vi "Regler Ausgang.vi"(7 "Index":i32, 8 "Fehler":errorcluster caption="Fehler (Eingang)") -> (0 "Fehler (Ausgang)":errorcluster)   [LabVIEW 2020, in "Regler.lvlib" / "Druckregler.lvlib"]
uses:
  Druckregler.lvlib
  Aktionen Param. Druckregler.ctl
  Aktionen Interne Werte.ctl
  Allgemein/FGV Zustaende Aktionen.ctl
  Funktionstasten/Zustaende.ctl
  Allgemein/Aktionen FGV Dichtheitstest.ctl
  Allgemein/Aktion FGV Messbetrieb.ctl
  Verwaltung/FGV IN Aktionen.ctl
  Konfig-Dateien/FGV Betriebsdaten Aktionen.ctl
  Verwaltung/Verwaltung - cRIO.lvlib
  Allgemein/Allgemein.lvlib
  Konfig-Dateien/Konfig-Dateien.lvlib
  Regler.lvlib
  Funktionstasten/Funktionstasten.lvlib
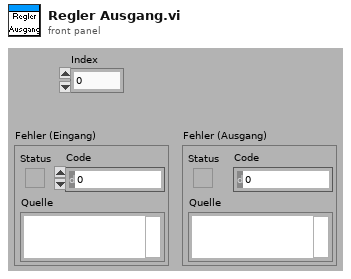
[diagram p1: front panel]
types:
  T1 = typedef "Allgemein.lvlib/Aktion FGV Messbetrieb.ctl" = enum16{"lesen", "schreiben"}
  T2 = typedef "Allgemein.lvlib/Aktionen FGV Dichtheitstest.ctl" = enum16{"lesen", "schreiben"}
  T3 = typedef "Funktionstasten.lvlib/Zustaende.ctl" = enum16{"Standby", "Pause", "Eco", "Messen", "Kalibrieren", "Spülen Filter", "Spülen Leitung", "Umgebungsluft", "0-Gas", "Cal-Gas", "CG zu PNS", "-------------", "Init 1", "Init 2", "Init 3", "Init 4", "Messen vorbereiten", "Messen durchführen", "Exit"}
  T4 = enum16{"Standby", "Pause", "Eco", "Messen", "Kalibrieren", "Spülen Filter", "Spülen Leitung", "Umgebungsluft", "0-Gas", "Cal-Gas 1", "CG zu PNS", "-------------", "Init 1", "Init 2", "Init 3", "Init 4", "Messen vorbereiten", "Messen durchführen", "Exit"}
  T5 = typedef "Allgemein.lvlib/FGV Zustaende Aktionen.ctl" = enum16{"lesen", "Zustand PC", "Zustand cRIO", "Bildnummer", "Samplepoint", "Sysloglevel"}
  T6 = typedef "Regler.lvlib/Druckregler.lvlib/Aktionen Interne Werte.ctl" = enum16{"lesen", "FT-IR", "Ausgang", "Pumpe", "laden", "speichern", "Änderung?", "Druck Kalter Block", "Dichtheitstest"}
  T7 = typedef "Regler.lvlib/Druckregler.lvlib/Aktionen Param. Druckregler.ctl" = enum16{"lesen", "schreiben", "Regler FT-IR", "Regler Ausgang", "Regler Durchfluss", "Regler PMA", "Regler NDIR", "Regler Filterblock", "Regler Gaskühler", "Regler Kalter Block"}
  T8 = typedef "Verwaltung - cRIO.lvlib/FGV IN Aktionen.ctl" = enum16{"lesen", "DI", "AI", "Fühler Br.", "TC", "Fühler Br. TC"}
  T9 = typedef "Konfig-Dateien.lvlib/FGV Betriebsdaten Aktionen.ctl" = enum16{"lesen", "Anlagengrenzw.", "PID Param.", "Sonstige", "Sensor Para."}
  T10 = typedef "Verwaltung - cRIO.lvlib/Analog Eingaenge.ctl" = cluster{"AI0: Durchfluss FT-IR":sgl, "AI1: Druck Ausgang":sgl, "AI2: Umgebungsdruck":sgl, "AI3: Druck FT-IR":sgl, "AI4: Druck CalGas":sgl, "AI5: Reserve":sgl, "AI6: Reserve":sgl, "AI7: Reserve":sgl, "Rohwert Durchfluss FT-IR":sgl, "Rohwert Druck Ausgang":sgl, "Rohwert Umgebungsdruck":sgl, "Rohwert Druck FT-IR":sgl, "Rohwert Druck CalGas":sgl, "Rohwert AI5":sgl, "Rohwert AI6":sgl, "Rohwert AI7":sgl, "Rohwert Diffdruck mbar FTIR":sgl}
  T11 = typedef "Anlagengrenzwerte.lvlib/Anlagen-Grenzwerte Anzeige.ctl" = cluster{"Eingangsdruck FT-IR:":T12, "Durchfluss FT-IR:":T12, "Durchfluss CalGas:":T12, "Druck Ausgang:":T12, "Druck Kalter Block:":T12, "Heizleitungen intern:":T12, "Heizleitung zu FT-IR:":T12, "Heizung Filterblock:":T12, "Heizung Pumpe:":T12, "Heizleitung Extern SP1:":T12, "Heizleitung Extern SP2:":T12, "FT-IR Heizung Messzelle:":T12, "Schaltschranktemperatur:":T12, "Gaskühler:":T12}
  T12 = typedef "Anlagengrenzwerte.lvlib/Anlagen-Parameter Anzeige.ctl" = cluster{"Sollwert":sgl, "Warn-Min":sgl, "Warn-Max":sgl, "Abschalt-Min":sgl, "Abschalt-Max":sgl, "Regler":u16}
  T13 = cluster{"Numerisch":sgl, "Numerisch":sgl, "Numerisch":sgl, "Numerisch":sgl, "Numerisch":sgl}
  T14 = typedef "Regler.lvlib/Druckregler.lvlib/Regler Interne Werte.ctl" = cluster{"PV":sgl, "D-action":sgl, "Error":sgl, "I-action":sgl, "OUT":sgl}
  T15 = typedef "Erweiterte Konfig.lvlib/Aktionen Dichtheitstest.ctl" = enum16{"Initialisieren", "Unterdruck aufbauen", "Prop schließen", "Warten", "Auswertung", "Fertig"}
  T16 = typedef "EPA 1065.lvlib/Dichtheitstest 1065-345.lvlib/Aktion Leak check durchfuehren.ctl" = enum16{"initialisieren", "Unterdruck erzeugen", "Ventile schließen", "Warten", "Auswertung", "fertig", "PDF erstellen", "abbrechen"}
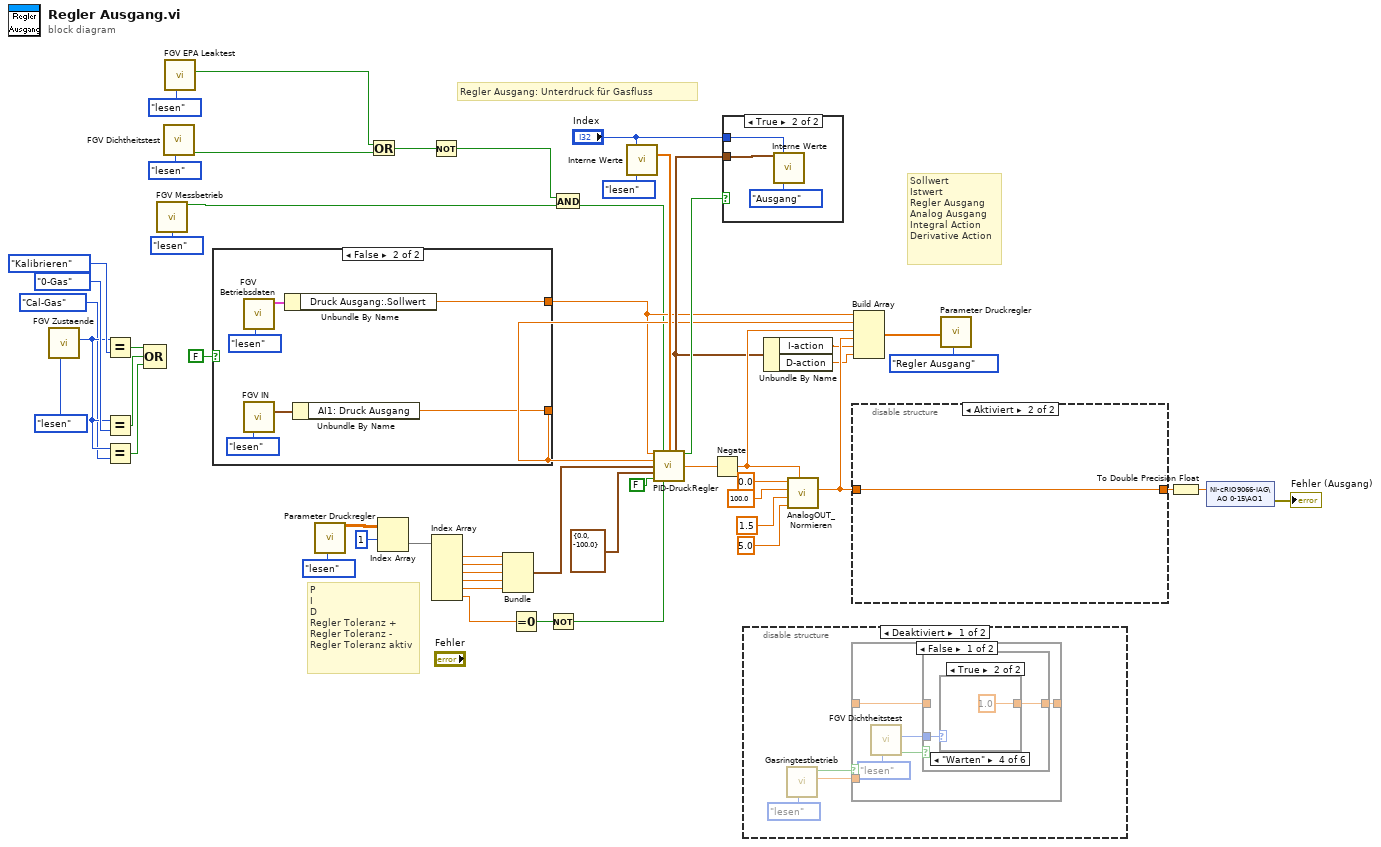
[diagram p0: block diagram]
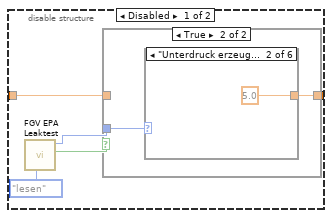
[diagram p2: hidden frame]
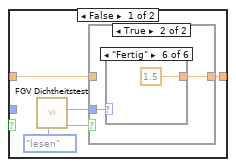
[diagram p3: hidden frame]
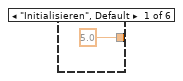
[diagram p5: hidden frame]
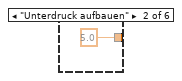
[diagram p6: hidden frame]
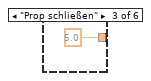
[diagram p7: hidden frame]
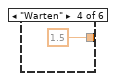
[diagram p8: hidden frame]
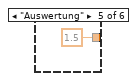
[diagram p9: hidden frame]
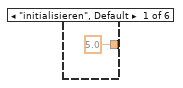
[diagram p10: hidden frame]
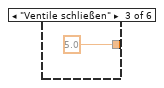
[diagram p11: hidden frame]
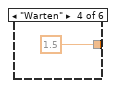
[diagram p12: hidden frame]
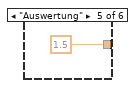
[diagram p13: hidden frame]
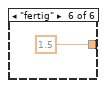
[diagram p14: hidden frame]
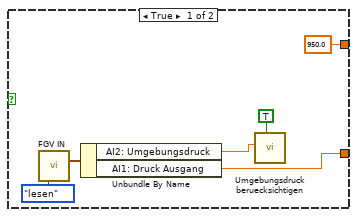
[diagram p15: hidden frame]
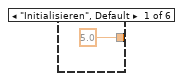
[diagram p17: hidden frame]
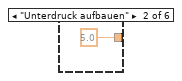
[diagram p18: hidden frame]
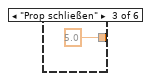
[diagram p19: hidden frame]
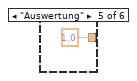
[diagram p20: hidden frame]
diagram:
  # "Regler Ausgang: Unterdruck für Gasfluss"
  # "Sollwert\nIstwert\nRegler Ausgang\nAnalog Ausgang\nIntegral Action\nDerivative Action"
  # "P\nI\nD\nRegler Toleranz +\nRegler Toleranz -\nRegler Toleranz aktiv"
  n1 = call "FGV Zustaende.vi"("Aktionen"=FGV_Zustaende_Aktionen."lesen") -> ("Zustand cRIO"=w16:T3)  [unwired: 6 in, 4 out]
  n2 = Equal?(x=w16, y=T4."Kalibrieren") -> (x = y?=w15:bool)
  n3 = Equal?(x=w16, y=T4."0-Gas") -> (x = y?=w14:bool)
  n4 = Equal?(x=w16, y=Zustaende."Cal-Gas") -> (x = y?=w13:bool)
  n5 = Compound Arithmetic op=OR ("Mehrfacharithmetik")(w15, w14, w13) -> ()  [unwired: 1 out]
  n6 = call "FGV Messbetrieb.vi"("Aktion"=Aktion_FGV_Messbetrieb."lesen") -> ("messen"=w1:bool)  [unwired: 13 in, 1 out]
  n7 = call "FGV Dichtheitstest.vi"("Aktionen"=Aktionen_FGV_Dichtheitstest."lesen") -> ("Dichtheitstest?"=w8:bool)  [unwired: 9 in, 1 out]
  n8 = call "FGV EPA Leaktest.vi"("Aktion"=enum16{"lesen", "schreiben"}."lesen") -> ("Leaktest aktiv"=w6:bool)  [unwired: 9 in, 1 out]
  n9 = case shown="False" FALSE {
    tunnel: [w58 w64] -> w22
    tunnel: [sgl 950.0 ("Sollwert") w61] -> w20
    frame True {
      n10 = call "FGV IN.vi"("Aktion"=FGV_IN_Aktionen."lesen") -> ("Analog Eingänge"=w59:T10)  [unwired: 10 in, 4 out]
      n11 = Unbundle By Name(w59) -> ("AI2: Umgebungsdruck"=w57:sgl, "AI1: Druck Ausgang"=w58:sgl)
      n12 = call "Umgebungsdruck beruecksichtigen.vi"("CalGas"=TRUE, "Umgebungsdruck"=w57) -> ()  [unwired: 9 in, 1 out]
    }
    frame False {
      n13 = call "FGV Betriebsdaten.vi"("Aktionen"=FGV_Betriebsdaten_Aktionen."lesen") -> ("Anlagen-Grenzwerte"=w62:T11)  [unwired: 7 in, 3 out]
      n14 = call "FGV IN.vi"("Aktion"=FGV_IN_Aktionen."lesen") -> ("Analog Eingänge"=w65:T10)  [unwired: 10 in, 4 out]
      n15 = Unbundle By Name(w62) -> ("Druck Ausgang:.Sollwert"=w61:sgl)
      n16 = Unbundle By Name(w65) -> ("AI1: Druck Ausgang"=w64:sgl)
    }
  }
  n17 = call "Parameter Druckregler.vi"("Aktionen"=Aktionen_Param._Druckregler."lesen") -> ("Regleparameter"=w39:sgl[][])  [unwired: 10 in, 8 out]
  n18 = Or(x=w6, y=w8) -> (x .or. y?=w4:bool)
  n19 = Index Array(array=w39, index (row)=1 ("Deaktivierter Index (Spalte)")) -> (element=w38:sgl[])  [unwired: 1 in]
  n20 = Not(x=w4) -> (.not. x?=w3:bool)
  n21 = Index Array(array=w38) -> (element #1=w50:sgl, element #2=w49:sgl, element #3=w48:sgl, element #4=w47:sgl, element #5=w46:sgl, element #6=w32:sgl)  [unwired: 6 in]
  n22 = Bundle("Numerisch"=w50, "Numerisch"=w49, "Numerisch"=w48, "Numerisch"=w47, "Numerisch"=w46) -> (w45:T13)  [unwired: 1 in]
  n23 = Equal To 0?(x=w32) -> (x = 0?=w44:bool)
  n24 = Not(x=w44) -> (.not. x?=w43:bool)
  n25 = And(x=w3, y=w1) -> (x .and. y?=w5:bool)
  n26 = call "Interne Werte.vi"("Index"="Index", "Aktionen Interne Werte"=Aktionen_Interne_Werte."lesen") -> ("Ausgang"=w30:sgl[])  [unwired: 7 in, 6 out]
  n27 = call "PID-DruckRegler.vi"("Sollwert"=w20, "Regler EIN"=w5, "Regler Interne Werte"=w30, "Istwert"=w22, "PID-Parameter"=w45, "output range"=cluster{"output high":sgl, "output low":sgl} {"output high"=0.0, "output low"=-100.0}, "Dichtheitstest"=FALSE, "Regler Toleranz verwenden?"=w43) -> ("Regler Interne Werte"=w26:T14, "Interne Werte speichern"=w27:bool, "Output"=w28:sgl)  [unwired: 5 in]
  n28 = Negate(x=w28) -> (-x=w35:sgl)
  n29 = case shown="True" w27 {
    tunnel: "Index" -> [_ w68]
    tunnel: w26 -> [_ w67]
    frame False {
    }
    frame True {
      n30 = call "Interne Werte.vi"("Regler Interne Werte"=w67, "Index"=w68, "Aktionen Interne Werte"=Aktionen_Interne_Werte."Ausgang") -> ()  [unwired: 6 in, 7 out]
    }
  }
  n31 = disable-structure shown="Deaktiviert" {
    frame Disabled {
      n32 = call "Gasringtestbetrieb.vi"("Aktion"=enum16{"lesen", "schreiben"}."lesen") -> ("Speed"=w72:dbl, "Manuell"=w71:bool)  [unwired: 9 in]
      n33 = case shown="False" w71 {
        tunnel: _ -> [w74 _]
        tunnel: [w73 w87] -> _
        tunnel: w72 -> [_ w87]
        frame False {
          n34 = call "FGV Dichtheitstest.vi"("Aktionen"=Aktionen_FGV_Dichtheitstest."lesen") -> ("Dichtheitstest?"=w75:bool, "Aktionen Dichtheitstest"=w76:T15)  [unwired: 9 in]
          n35 = case shown="True" w75 {
            tunnel: w76 -> [_ w80]
            tunnel: w74 -> [w78 _]
            tunnel: [w78 w79] -> w73
            frame False {
            }
            frame True {
              n36 = case shown="\"Warten\"" w80 {
                tunnel: [sgl 5.0 ("Untergrenze") sgl 5.0 ("Untergrenze") sgl 5.0 ("Untergrenze") sgl 1.0 ("Untergrenze") sgl 1.0 ("Untergrenze") sgl 1.0 ("Untergrenze")] -> w79
                frame "Initialisieren", Default {
                }
                frame "Unterdruck aufbauen" {
                }
                frame "Prop schließen" {
                }
                frame "Warten" {
                }
                frame "Auswertung" {
                }
                frame "Fertig" {
                }
              }
            }
          }
        }
        frame True {
        }
      }
    }
    frame Enabled {
    }
  }
  n37 = Unbundle By Name(w26) -> ("I-action"=w25:sgl, "D-action"=w24:sgl)
  n38 = call "AnalogOUT_Normieren.vi"("Analogwert"=w35, "Obergrenze"=sgl 5.0, "Untergrenze"=sgl 1.5, "Max Analogwert"=sgl 100.0, "Min Analogwert"=sgl 0.0) -> ("Normierter Wert"=w33:sgl)  [unwired: 6 in]
  n39 = disable-structure shown="Aktiviert" {
    disable-tunnel: w33 -> [w92 w115]
    disable-tunnel: [w91 w115] -> w21
    frame Disabled {
      n40 = call "FGV EPA Leaktest.vi"("Aktion"=enum16{"lesen", "schreiben"}."lesen") -> ("Leaktest aktiv"=w89:bool, "Leaktest Zustand"=w88:T16)  [unwired: 9 in]
      n41 = case shown="True" w89 {
        tunnel: w92 -> [w97 _]
        tunnel: [w96 w108] -> w91
        tunnel: w88 -> [_ w107]
        frame False {
          n42 = call "FGV Dichtheitstest.vi"("Aktionen"=Aktionen_FGV_Dichtheitstest."lesen") -> ("Dichtheitstest?"=w93:bool, "Aktionen Dichtheitstest"=w94:T15)  [unwired: 9 in]
          n43 = case shown="True" w93 {
            tunnel: w94 -> [_ w100]
            tunnel: w97 -> [w98 _]
            tunnel: [w98 w99] -> w96
            frame False {
            }
            frame True {
              n44 = case shown="\"Fertig\"" w100 {
                tunnel: [sgl 5.0 ("Untergrenze") sgl 5.0 ("Untergrenze") sgl 5.0 ("Untergrenze") sgl 1.5 ("Untergrenze") sgl 1.5 ("Untergrenze") sgl 1.5 ("Untergrenze")] -> w99
                frame "Initialisieren", Default {
                }
                frame "Unterdruck aufbauen" {
                }
                frame "Prop schließen" {
                }
                frame "Warten" {
                }
                frame "Auswertung" {
                }
                frame "Fertig" {
                }
              }
            }
          }
        }
        frame True {
          n45 = case shown="\"Unterdruck erzeugen\"" w107 {
            tunnel: [sgl 5.0 ("Untergrenze") sgl 5.0 ("Untergrenze") sgl 5.0 ("Untergrenze") sgl 1.5 ("Untergrenze") sgl 1.5 ("Untergrenze") sgl 1.5 ("Untergrenze")] -> w108
            frame "initialisieren", Default {
            }
            frame "Unterdruck erzeugen" {
            }
            frame "Ventile schließen" {
            }
            frame "Warten" {
            }
            frame "Auswertung" {
            }
            frame "fertig" {
            }
          }
        }
      }
    }
    frame Enabled {
    }
  }
  n46 = Build Array(w20, w22, w35, w33, w25, w24) -> (w41:sgl[])
  n47 = call "Parameter Druckregler.vi"("Werte Ausgang"=w41, "Aktionen"=Aktionen_Param._Druckregler."Regler Ausgang") -> ()  [unwired: 9 in, 9 out]
  n48 = To Double Precision Float(number=w21) -> (double precision float=w34:dbl)
  n49 = shared-variable "NI-cRIO9066-IAG\\AO 0-15\\AO1"(w34) -> (error out=→"Fehler (Ausgang)":errorcluster)  [unwired: 1 in]
